vi "drawpicture.vi"(9 "y":cluster{"left":i16, "top":i16}, 10 "2D Picture":picture, 11 "name or relative path":path) -> (3 "new picture":picture)   [LabVIEW 2025]
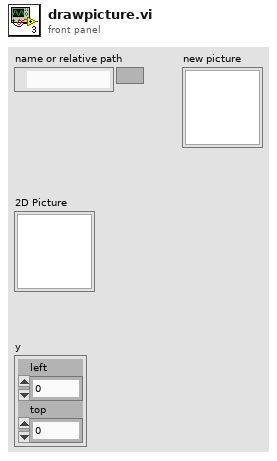
[diagram p1: front panel]
types:
  T1 = typedef "imagedata.ctl" = cluster{"image type":i32, "image depth":i32, "image":u8[], "mask":u8[], "colors":u32[], "Rectangle":cluster{"left":i16, "top":i16, "right":i16, "bottom":i16}}
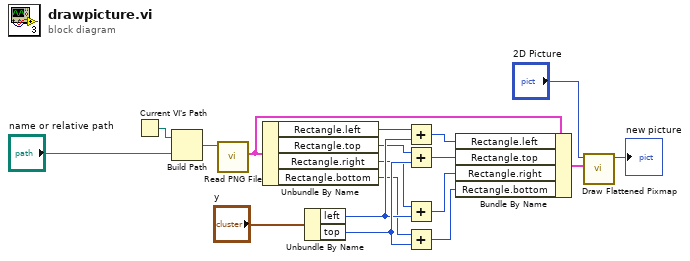
[diagram p0: block diagram]
diagram:
  n1 = Current VI's Path() -> (path=w1:path)
  n2 = Build Path(base path=w1, name or relative path="name or relative path") -> (appended path=w3:path)
  n3 = call <vilib>:"Read PNG File.vi"("path to PNG file"=w3) -> ("image data"=w13:T1)  [unwired: 8 in, 2 out]
  n4 = Unbundle By Name(w13) -> ("Rectangle.left"=w7:i16, "Rectangle.top"=w8:i16, "Rectangle.right"=w9:i16, "Rectangle.bottom"=w10:i16)
  n5 = Unbundle By Name("y") -> ("left"=w11:i16, "top"=w12:i16)
  n6 = Add(x=w7, y=w11) -> (x+y=w14:i16)
  n7 = Add(x=w8, y=w12) -> (x+y=w15:i16)
  n8 = Add(x=w9, y=w11) -> (x+y=w16:i16)
  n9 = Add(x=w10, y=w12) -> (x+y=w17:i16)
  n10 = Bundle By Name(cluster=w13, "Rectangle.left"=w14, "Rectangle.top"=w15, "Rectangle.right"=w16, "Rectangle.bottom"=w17) -> (w18:T1)
  n11 = call <vilib>:"Draw Flattened Pixmap.vi"("image data"=w18, "picture"="2D Picture") -> ("new picture"=→"new picture":picture)  [unwired: 7 in]
